vi "Host.vi"() -> ()   [LabVIEW 2015]
uses:
  <vilib>/NI Veristand/Execution/Workspace/NI VeriStand - Get Multiple Channel Values.vi
  <vilib>/NI Veristand/Execution/Workspace/NI VeriStand - Set Single Channel Value.vi
  <vilib>/NI Veristand/Execution/Project/NI_VS Project ExecutionAPI.lvlib
  <vilib>/NI Veristand/Execution/Workspace/NI_VS Workspace ExecutionAPI.lvlib
panel:
  in  "Trigger DMA":bool
  in  "Tab Control":enum32{"Table", "DMA Waveform"}(tab)
  out "Table":string[][](table)
  out "Graph":waveform(dbl)[](graph)
  in  "Exit":bool
  in  "Engine RPM":dbl
  in  "Crank Pattern":T1(ring)
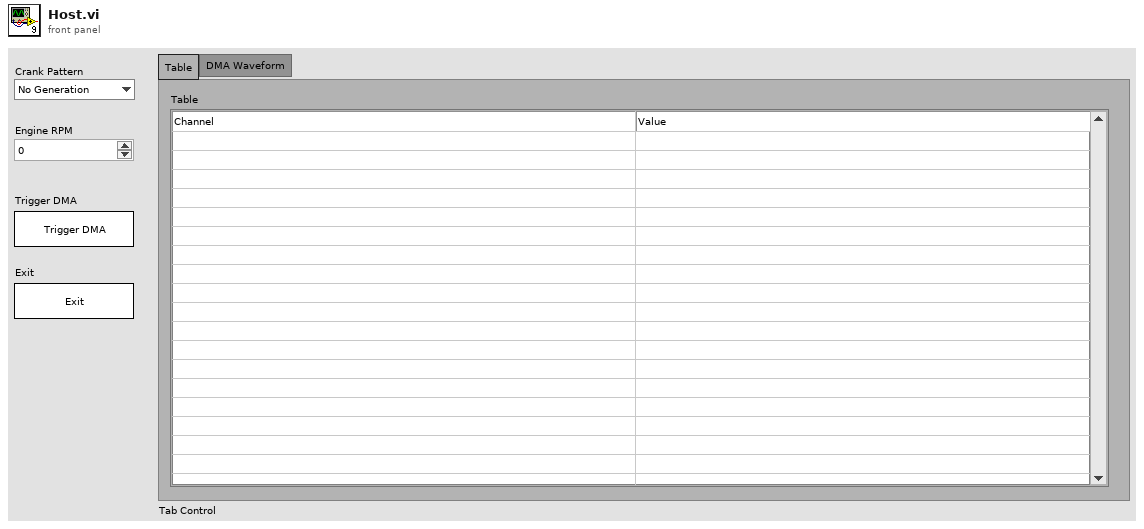
[diagram p1: front panel]
types:
  T1 = enum16{"No Generation", "Pattern 1", "Pattern 2"}
  T2 = typedef "NI_VS Project ExecutionAPI.lvlib/Project Ref.ctl" = refnum<k24>
  T3 = typedef "NI_VS Workspace ExecutionAPI.lvlib/WorkspaceAPI.ctl" = refnum<k24>
  T4 = typedef "NI_VS Workspace ExecutionAPI.lvlib/NodeInfo.ctl" = cluster{"Name":string, "FullPath":string, "Type":string, "IsChannel":bool, "Channel":cluster{"Unit":string, "Readable":bool, "Writable":bool, "Faultable":bool, "Scalable":bool, "RowDim":u32, "ColumnDim":u32, "Value Table Names":string[], "Value Table Values":dbl[]}, "IsWaveform":bool, "Waveform":cluster{"DataType":T5}}
  T5 = typedef "NI_VS Workspace ExecutionAPI.lvlib/Waveform Data Type.ctl" = enum16{"Double", "ComplexDouble"}
  T6 = typedef "NI_VS Waveform Streaming Interface.lvlib/WaveformStreamSpecification.ctl" = refnum<k24>
  T7 = typedef "NI_VS Waveform Streaming Interface.lvlib/Registered Waveform Streams Data Event Refnum (DBL).ctl" = cluster{"Callback Refnum":refnum<k27>, "Data Event":refnum<user-event>, "Event Refnum":refnum<event-registration>, "WaveformDataWatcherDBL":T8}
  T8 = typedef "NI_VS Waveform Streaming Interface.lvlib/WaveformDataWatcherDBL.ctl" = refnum<k24>
  T9 = typedef "NI_VS Waveform Streaming Interface.lvlib/WaveformStreamingAPI.ctl" = refnum<k24>
  T10 = cluster{"Waveform.Refs":T6[], "WaveformStreaming.Event.Refs":T7, "WaveformStreaming.Ref":T9}
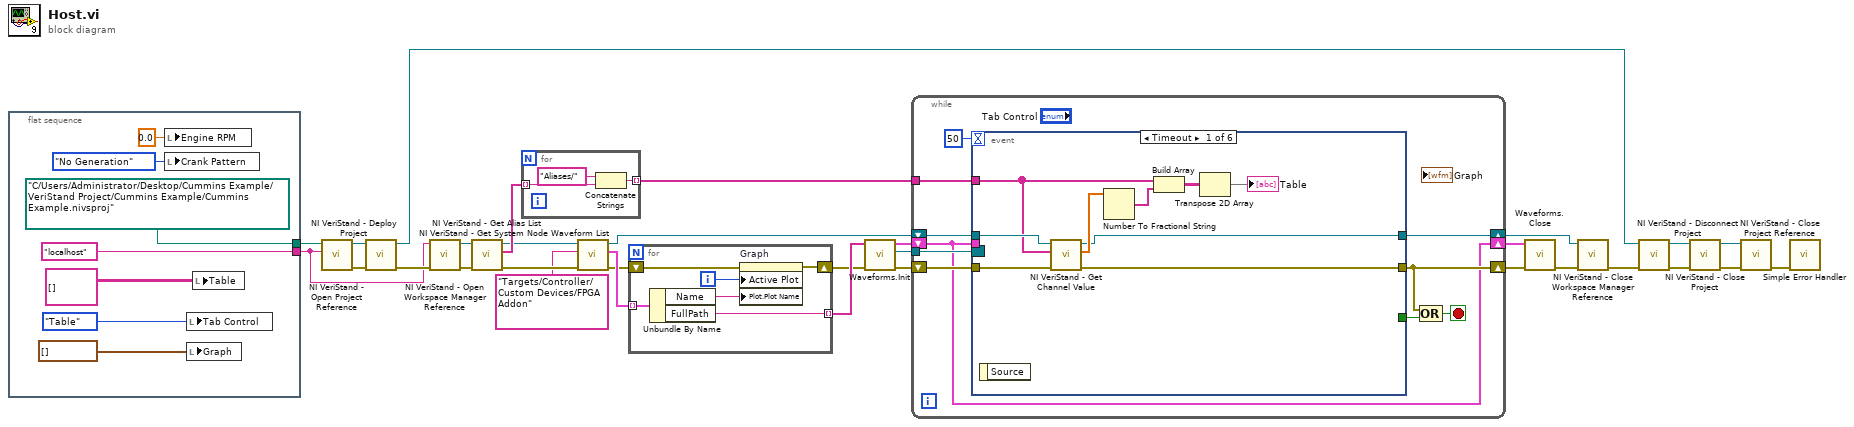
[diagram p0: block diagram]
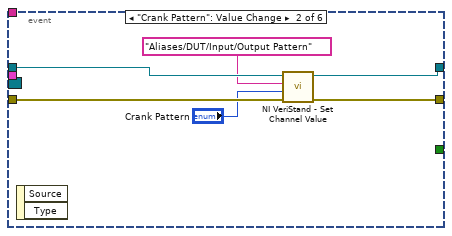
[diagram p2: hidden frame]
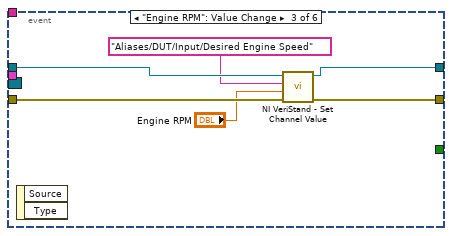
[diagram p3: hidden frame]
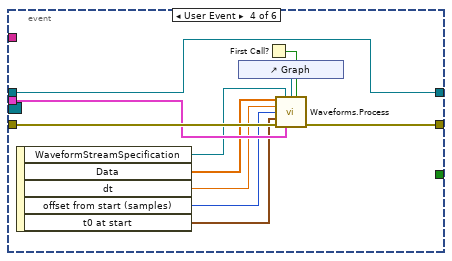
[diagram p4: hidden frame]
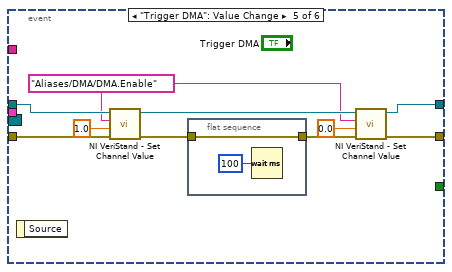
[diagram p5: hidden frame]
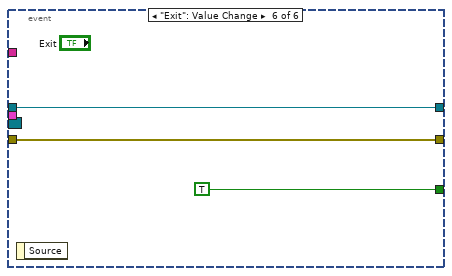
[diagram p6: hidden frame]
diagram:
  n1 = flat-sequence {
    tunnel: [path "C:/Users/Administrator/Desktop/Cummins Example/VeriStand Project/Cummins Example/Cummins Example.nivsproj" ("Project File Path")] -> w29
    tunnel: ["localhost" ("Gateway IP Address (\"\": localhost)")] -> w1
    frame #0 {
      n2 = local write "Engine RPM"(0.0 ("Engine RPM")) -> ()
      n3 = local write "Crank Pattern"(T1."No Generation" ("Crank Pattern")) -> ()
      n4 = local write "Tab Control"(enum32{"Table", "DMA Waveform"}."Table" ("Tab Control")) -> ()
      n5 = local write "Graph"(waveform(dbl)[] [] ("Graph")) -> ()
      n6 = local write "Table"(string[][] [] ("Table")) -> ()
    }
  }
  n7 = call <vilib>:"NI VeriStand - Open Project Reference.vi"("Gateway IP Address (\"\": localhost)"=w1, "Project File Path"=w29) -> ("error out"=w30:errorcluster, "Project Ref"=w31:T2)  [unwired: 8 in]
  n8 = call <vilib>:"NI VeriStand - Deploy Project.vi"("error in (no error)"=w30, "Project Ref in"=w31) -> ("error out"=w23:errorcluster, "Project Ref out"=w22:T2)  [unwired: 8 in]
  n9 = call <vilib>:"NI VeriStand - Open Workspace Manager Reference.vi"("error in (no error)"=w23, "Gateway IP Address (\"\": localhost)"=w1) -> ("error out"=w27:errorcluster, "WorkspaceManager"=w28:T3)  [unwired: 8 in]
  n10 = call <vilib>:"NI VeriStand - Get Alias List.vi"("error in (no error)"=w27, "WorkspaceManager in"=w28) -> ("error out"=w13:errorcluster, "Aliases"=w21:string[], "WorkspaceManager out"=w11:T3)  [unwired: 6 in, 1 out]
  n11 = for {
    tunnel: w21 -> [w41] mode=indexing
    tunnel: [w39] -> w20 mode=indexing
    n12 = Concatenate Strings("Aliases/" ("string"), w41) -> (w39:string)
  }
  n13 = call <vilib>:"NI VeriStand - Get System Node Waveform List.vi"("error in (no error)"=w13, "StartNode (\"\")"="Targets/Controller/Custom Devices/FPGA Addon" ("StartNode (\"\")"), "WorkspaceManager in"=w11) -> ("error out"=w2:errorcluster, "Waveforms"=w9:T4[], "WorkspaceManager out"=w10:T3)  [unwired: 6 in]
  n14 = for {
    tunnel: w9 -> [w47] mode=indexing
    tunnel: [w46] -> w8 mode=indexing
    shift-right: [w44] -> w3
    shift-left: w2 -> [w42]
    i -> [w43]
    n15 = Unbundle By Name(w47) -> ("Name"=w45:string, "FullPath"=w46:string)
    n16 = property on="Graph" class="WFGraph (strict)"(error in=w42, "Active Plot"=w43, "Plot.Plot Name"=w45) -> (error out=w44:errorcluster)  [unwired: 1 in, 1 out]
  }
  n17 = call "Waveforms.Init.vi"("error in"=w3, "Channel.Paths"=w8) -> ("error out"=w15:errorcluster, "WaveformStreaming.Event"=w14:refnum<event-registration>, "Waveforms"=w7:T10)  [unwired: 7 in]
  n18 = while {
    tunnel: w20 -> [w55]
    shift-right: [w53] -> w25
    shift-left: w10 -> [w56]
    shift-right: [w52] -> w5
    shift-left: w15 -> [w57]
    tunnel: w14 -> [w49]
    shift-right: [w48] -> w6
    shift-left: w7 -> [w48]
    stop <- w50 stop-if-true
    n19 = event shown="[0] Timeout" {
      selector: w49 -> [_ _ _ _ _ _]
      dyn-events: _ -> [_ _ _ _ _ _]
      timeout: 50 -> [_ _ _ _ _ _]
      tunnel: w57 -> [w66 w72 w78 w89 w99 w104]
      tunnel: w56 -> [w65 w71 w77 w80 w98 w103]
      tunnel: w55 -> [w61 _ _ _ _ _]
      tunnel: [w59 w69 w75 w80 w94 w103] -> w53
      tunnel: [w58 w70 w76 w82 w95 w104] -> w52
      tunnel: [_ _ _ _ _ TRUE] -> w51
      tunnel: w48 -> [_ _ _ w88 _ _]
      event Timeout {
        n20 = event-data() -> ()  [unwired: 1 in, 1 out]
        n21 = call-poly <vilib>:"NI VeriStand - Get Channel Value.vi"("error in (no error)"=w66, "Channels"=w61, "WorkspaceManager in"=w65) -> ("error out"=w58:errorcluster, "Values"=w62:dbl[], "WorkspaceManager out"=w59:T3)  [unwired: 6 in]
        n22 = Number To Fractional String(number=w62) -> (F-format string=w64:string[])  [unwired: 3 in]
        n23 = Build Array(w61, w64) -> (w63:string[][])
        n24 = Transpose 2D Array(2D array=w63) -> (transposed array=→"Table":string[][])
      }
      event "Crank Pattern": Value Change {
        n25 = event-data() -> ()  [unwired: 1 in, 2 out]
        n26 = call-poly <vilib>:"NI VeriStand - Set Channel Value.vi"("error in (no error)"=w72, "Value"="Crank Pattern", "Channel"="Aliases/DUT/Input/Output Pattern" ("string"), "WorkspaceManager in"=w71) -> ("error out"=w70:errorcluster, "WorkspaceManager out"=w69:T3)  [unwired: 6 in]
      }
      event "Engine RPM": Value Change {
        n27 = event-data() -> ()  [unwired: 1 in, 2 out]
        n28 = call-poly <vilib>:"NI VeriStand - Set Channel Value.vi"("error in (no error)"=w78, "Value"="Engine RPM", "Channel"="Aliases/DUT/Input/Desired Engine Speed" ("string"), "WorkspaceManager in"=w77) -> ("error out"=w76:errorcluster, "WorkspaceManager out"=w75:T3)  [unwired: 6 in]
      }
      event User Event {
        n29 = event-data() -> ("WaveformStreamSpecification"=w83:T6, "Data"=w87:dbl[], "dt"=w86:dbl, "offset from start (samples)"=w85:u64, "t0 at start"=w84:timestamp)  [unwired: 1 in]
        n30 = control-ref of="Graph"() -> (w81:refnum<vi>)
        n31 = First Call?() -> (First Call?: T/F=w79:bool)
        n32 = call "Waveforms.Process.vi"("Data"=w87, "Waveform.Ref"=w83, "WaveformGraph.Ref"=w81, "Reset?"=w79, "dt"=w86, "offset from start (samples)"=w85, "t0 at start"=w84, "error in (no error)"=w89, "Waveforms"=w88) -> ("error out"=w82:errorcluster)  [unwired: 6 in]
      }
      event "Trigger DMA": Value Change {
        w91 = "Aliases/DMA/DMA.Enable" ("string")
        n33 = event-data() -> ()  [unwired: 1 in, 1 out]
        n34 = call-poly <vilib>:"NI VeriStand - Set Channel Value.vi"("error in (no error)"=w99, "Value"=1.0, "Channel"=w91, "WorkspaceManager in"=w98) -> ("error out"=w92:errorcluster, "WorkspaceManager out"=w96:T3)  [unwired: 6 in]
        n35 = flat-sequence {
          tunnel: [w100] -> w93
          tunnel: w92 -> [w100]
          frame #0 {
            n36 = Wait (ms)(milliseconds to wait=u32 100) -> ()  [unwired: 1 out]
          }
        }
        n37 = call-poly <vilib>:"NI VeriStand - Set Channel Value.vi"("error in (no error)"=w93, "Value"=0.0, "Channel"=w91, "WorkspaceManager in"=w96) -> ("error out"=w95:errorcluster, "WorkspaceManager out"=w94:T3)  [unwired: 6 in]
      }
      event "Exit": Value Change {
        n38 = event-data() -> ()  [unwired: 1 in, 1 out]
      }
    }
    n39 = Compound Arithmetic op=OR(w52, w51) -> (w50:bool)
  }
  n40 = call "Waveforms.Close.vi"("error in (no error)"=w5, "Waveforms"=w6) -> ("error out"=w4:errorcluster)  [unwired: 9 in]
  n41 = call <vilib>:"NI VeriStand - Close Workspace Manager Reference.vi"("error in (no error)"=w4, "WorkspaceManager"=w25) -> ("error out"=w24:errorcluster)  [unwired: 9 in]
  n42 = call <vilib>:"NI VeriStand - Disconnect Project.vi"("error in (no error)"=w24, "Project Ref in"=w22) -> ("error out"=w18:errorcluster, "Project Ref out"=w26:T2)  [unwired: 8 in]
  n43 = call <vilib>:"NI VeriStand - Close Project.vi"("error in (no error)"=w18, "Project Ref in"=w26) -> ("error out"=w17:errorcluster, "Project Ref out"=w19:T2)  [unwired: 8 in]
  n44 = call <vilib>:"NI VeriStand - Close Project Reference.vi"("error in (no error)"=w17, "Project Ref"=w19) -> ("error out"=w16:errorcluster)  [unwired: 9 in]
  n45 = call <vilib>:"Simple Error Handler.vi"("error in (no error)"=w16) -> ()  [unwired: 4 in, 5 out]
